vi "Write Channel Names.vi"(8 "error in (no error)":errorcluster, 10 "Channel Names":string[](array[string]), 11 "Analog-Output in":refnum<class "Analog-Output.lvclass">) -> (0 "error out":errorcluster, 3 "Analog-Output out":refnum<class "Analog-Output.lvclass">)   [LabVIEW 2019, in "Analog-Output.lvlib" / "Analog-Output.lvclass"]
uses:
  Library/Analog-Output.lvclass
  Library/Analog-Output.lvclass/Analog-Output.ctl
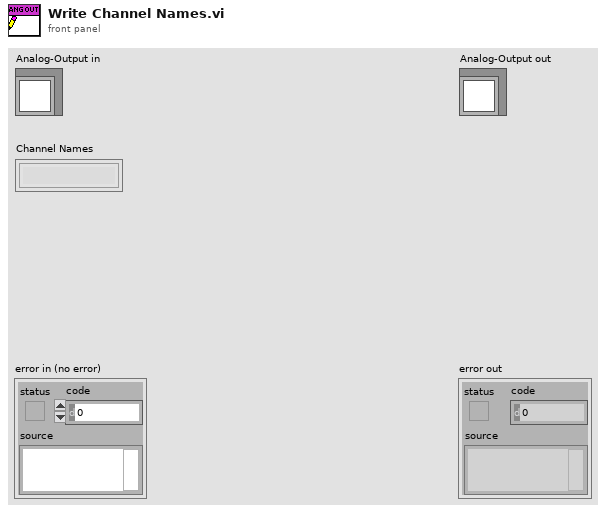
[diagram p1: front panel]
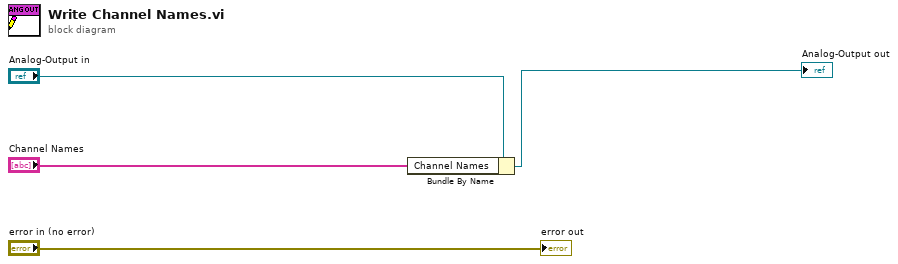
[diagram p0: block diagram]
diagram:
  n1 = Bundle By Name(cluster="Analog-Output in", "Channel Names"="Channel Names") -> (→"Analog-Output out":refnum<class "Analog-Output.lvclass">)
  "error out" <- "error in (no error)"
